vi "while loop.vi"() -> ()   [LabVIEW 2012]
panel:
  out "Array 2":dbl[](array[numeric])
  out "Array":dbl[](array[numeric])
  out "Waveform Graph":cluster{dbl, dbl, dbl[]}(graph)
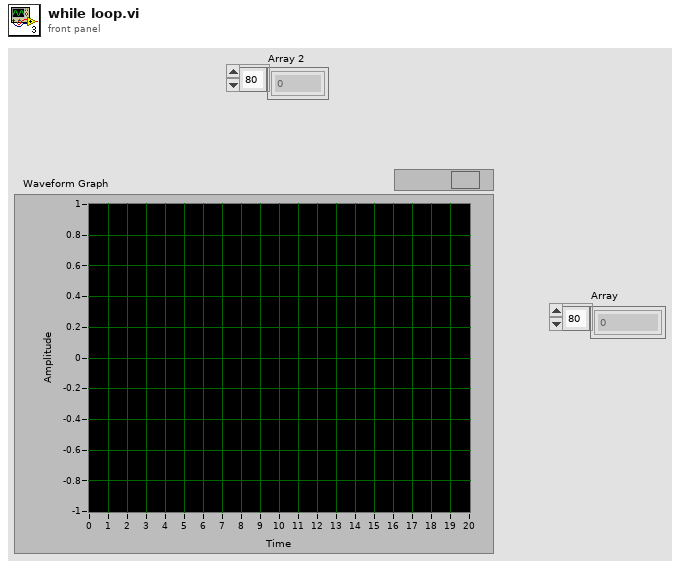
[diagram p1: front panel]
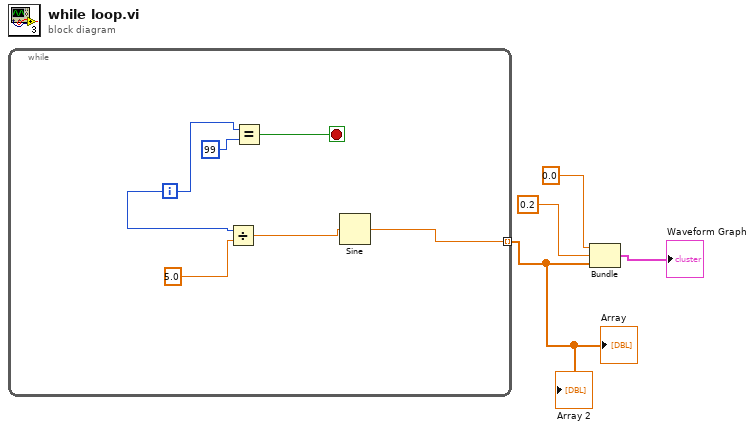
[diagram p0: block diagram]
diagram:
  n1 = while {
    tunnel: [w9] -> w1 mode=indexing
    i -> [w6]
    stop <- w5 stop-if-true
    n2 = Divide(x=w6, y=5.0) -> (x/y=w10:dbl)
    n3 = Equal?(x=w6, y=99) -> (x = y?=w5:bool)
    n4 = Sine(x=w10) -> (sin(x)=w9:dbl)
  }
  "Array" <- w1
  "Array 2" <- w1
  n5 = Bundle(0.0, 0.2, w1) -> (→"Waveform Graph":cluster{dbl, dbl, dbl[]})  [unwired: 1 in]
